vi "CALC_TRAN_TIME_STEP_RTIM.vi"(0 "VISA IN":refnum<visa-resource-name>, 1 "Rise Time(sec)":i32, 5 "error in":errorcluster, 7 "Channel":i32) -> (14 "VISA Out":refnum<visa-resource-name>, 19 "error out":errorcluster)   [LabVIEW 2018, in "PNA-X.lvlib"]
doc: "CALCulate<cnum>:TRANsform:TIME:STEP:RTIMe <num> \n(Read-Write) Sets the step rise time for the transform window. \nSee Critical Note \nParameters \n<cnum> Channel number of the measurement. There must be a selected measurement \non that channel. If unspecified, <cnum> is set to 1. \n<num> Rise time in seconds; Choose any number between: \n.45 / frequency span and 1.48 / frequency span \nExamples CALC:TRAN:TIME:STEP:RTIM 1e-8 \ncalculate2:transform:time:step:rtime 15 ps \nQuery Syntax CALCulate<cnum>:TRANsform:TIME:STEP:RTIMe? \nReturn Type Numeric \nDefault .99 / Default Span"
uses:
  PNA-X.lvlib
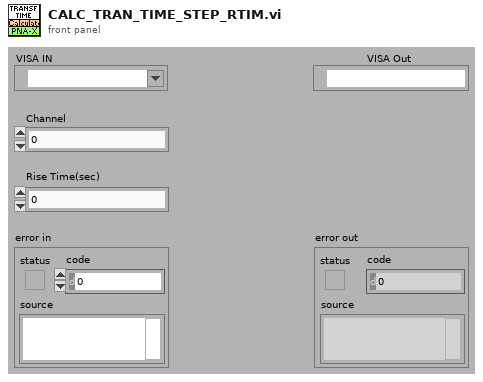
[diagram p1: front panel]
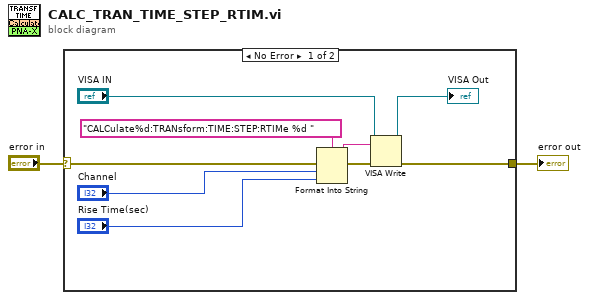
[diagram p0: block diagram]
diagram:
  n1 = case shown="No Error" "error in" {
    selector: "error in" -> [w11 w12]
    tunnel: [w6 w12] -> w1
    frame No Error {
      n2 = Format Into String(format string="CALCulate%d:TRANsform:TIME:STEP:RTIMe %d " ("Cmdline"), error in=w11, "Channel", "Rise Time(sec)") -> (resulting string=w9:string, error out=w10:errorcluster)  [unwired: 1 in]
      n3 = VISA Write(VISA resource name="VISA IN", write buffer=w9, error in (no error)=w10) -> (VISA resource name out=→"VISA Out":refnum<visa-resource-name>, error out=w6:errorcluster)  [unwired: 1 out]
    }
    frame Error {
    }
  }
  "error out" <- w1
